vi "Salidas.vi"(11 "Class 2.lvclass":refnum<class "Class 2.lvclass">) -> (3 "Class 2.lvclass 2":refnum<class "Class 2.lvclass">)   [LabVIEW 2019, in "Class 2.lvclass"]
uses:
  Class 2.lvclass
  Class 2.lvclass/Class 2.ctl
  Datos Out.vi
panel:
  out "MAQ DE ESTADOS":T1
  out "SALIDAS.SMAC DISTANCIA":dbl
  out "SALIDAS.SMAC g":dbl
  out "SALIDAS.MENSAJES":string
  out "SALIDAS.SAMAC AVANZANDO":bool
  out "SALIDAS.SEMAC RETORNANDO":bool
  out "SALIDAS.CILINDRO 2":bool
  out "SALIDAS.CILINDRO 1":bool
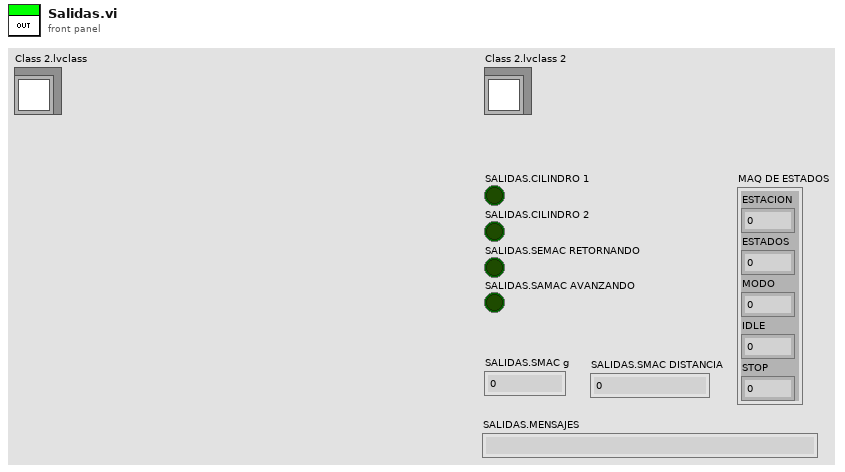
[diagram p1: front panel]
types:
  T1 = cluster{"ESTACION":i32, "ESTADOS":i16, "MODO":i16, "IDLE":i16, "STOP":i16}
  T2 = cluster{"SALIDAS.CILINDRO 1":bool, "SALIDAS.CILINDRO 2":bool, "SALIDAS.SEMAC RETORNANDO":bool, "SALIDAS.SAMAC AVANZANDO":bool, "Auto(off)/Manual(on)":bool, "HOME_CILINDRO_1":bool, "HOME_CILINDRO_2":bool, "AVANCE_CILINDRO_1":bool, "AVANCE_CILINDRO_2":bool, "PIEZA_EN_NIDO":bool, "BIMANUAL 2":bool, "BIMANUAL1":bool, "SIN CAMBIOS":bool, "CON  CAMBIOS":bool, "TESTER":bool, "MAQUINA EN ORIGEN":bool, "FALLA PRESENTE":bool}
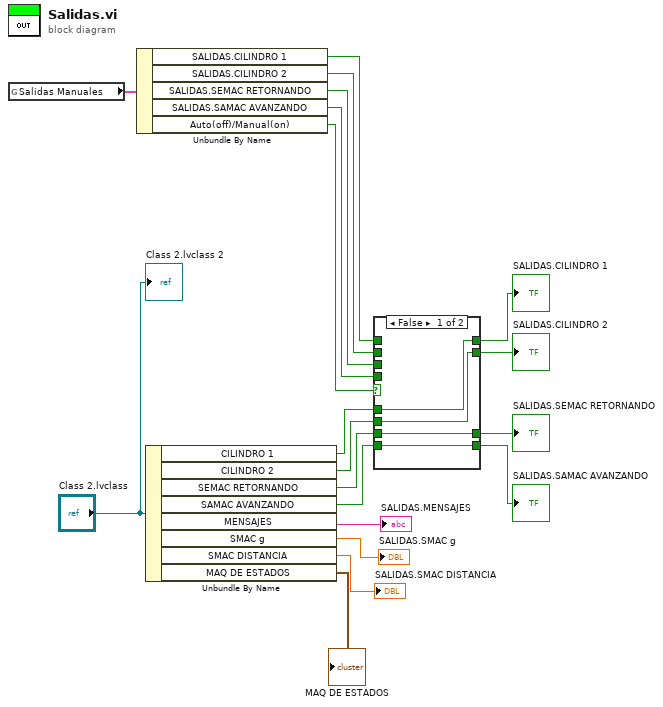
[diagram p0: block diagram]
diagram:
  n1 = global read "Datos Out.vi" "Salidas Manuales"() -> (w1:T2)
  n2 = Unbundle By Name(w1) -> ("SALIDAS.CILINDRO 1"=w14:bool, "SALIDAS.CILINDRO 2"=w13:bool, "SALIDAS.SEMAC RETORNANDO"=w12:bool, "SALIDAS.SAMAC AVANZANDO"=w11:bool, "Auto(off)/Manual(on)"=w15:bool)
  n3 = Unbundle By Name("Class 2.lvclass") -> ("CILINDRO 1"=w10:bool, "CILINDRO 2"=w9:bool, "SEMAC RETORNANDO"=w8:bool, "SAMAC AVANZANDO"=w7:bool, "MENSAJES"=→"SALIDAS.MENSAJES":string, "SMAC g"=→"SALIDAS.SMAC g":dbl, "SMAC DISTANCIA"=→"SALIDAS.SMAC DISTANCIA":dbl, "MAQ DE ESTADOS"=→"MAQ DE ESTADOS":T1)
  n4 = case shown="False" w15 {
    tunnel: w14 -> [_ w27]
    tunnel: w13 -> [_ w26]
    tunnel: w12 -> [_ w25]
    tunnel: w11 -> [_ w24]
    tunnel: w10 -> [w23 _]
    tunnel: w9 -> [w22 _]
    tunnel: w8 -> [w21 _]
    tunnel: w7 -> [w20 _]
    tunnel: [w23 w27] -> w6
    tunnel: [w22 w26] -> w5
    tunnel: [w21 w25] -> w4
    tunnel: [w20 w24] -> w3
    frame False {
    }
    frame True {
    }
  }
  "SALIDAS.CILINDRO 1" <- w6
  "SALIDAS.CILINDRO 2" <- w5
  "SALIDAS.SEMAC RETORNANDO" <- w4
  "SALIDAS.SAMAC AVANZANDO" <- w3
  "Class 2.lvclass 2" <- "Class 2.lvclass"
